vi "Initialize Channel Browser_Trigger.vi"(8 "error in (no error)":errorcluster, 9 "Trigger Parameters":T1, 10 ".NET Refnum in":refnum<k24>, 11 "Item Ref in":T2 format="%.0x") -> (0 "error out":errorcluster, 2 "Event":refnum<user-event>, 3 "Item Ref out":T2 format="%.0x")   [LabVIEW 2018, in "Instrument Addon System Explorer.lvlib"]
uses:
  Instrument Addon System Explorer.lvlib
  <vilib>/NI VeriStand/Custom Device Tools/Custom Device Utility Library/Custom Device Utility Library.lvlib
  <vilib>/NI VeriStand/Custom Device API/Custom Device API.lvlib
  NationalInstruments.VeriStand.SystemStorage
  NationalInstruments.VeriStand.SystemStorageUI
  <vilib>/NI VeriStand/UI Controls/Single Node Browser/NI_VS UI Single Node Browser.lvlib
  NationalInstruments.VeriStand
  Addon Shared/SubVIs/Constants.vi
  Addon Shared/Instrument Addon Shared.lvlib
  <vilib>/NI VeriStand/Custom Device API/Custom Device Item Ref.ctl
  <vilib>/NI VeriStand/UI Controls/Single Node Browser/Net Event.ctl
  <vilib>/NI VeriStand/UI Controls/Single Node Browser/Net Event Data.ctl
  Addon Shared/Types/Trigger Parameters.ctl
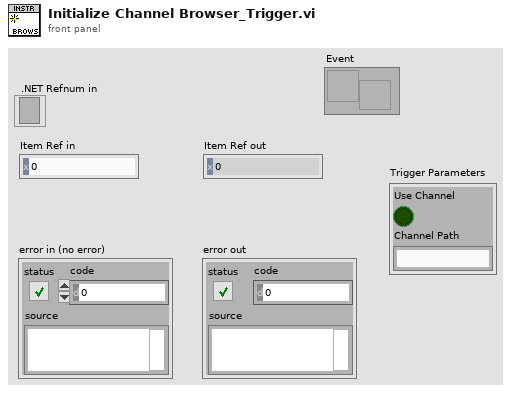
[diagram p1: front panel]
types:
  T1 = typedef "Instrument Addon Shared.lvlib/Trigger Parameters.ctl" = cluster{"Use Channel":bool, "Channel Path":string}
  T2 = typedef "Custom Device API.lvlib/Custom Device Item Ref.ctl" = u64
  T3 = typedef "Custom Device API.lvlib/Custom Device Pointer.ctl" = refnum<k24>
  T4 = typedef "NI_VS UI Single Node Browser.lvlib/Callback Type.ctl" = cluster{"Net Callbacks":refnum<k27>[], "Event":refnum<user-event>}
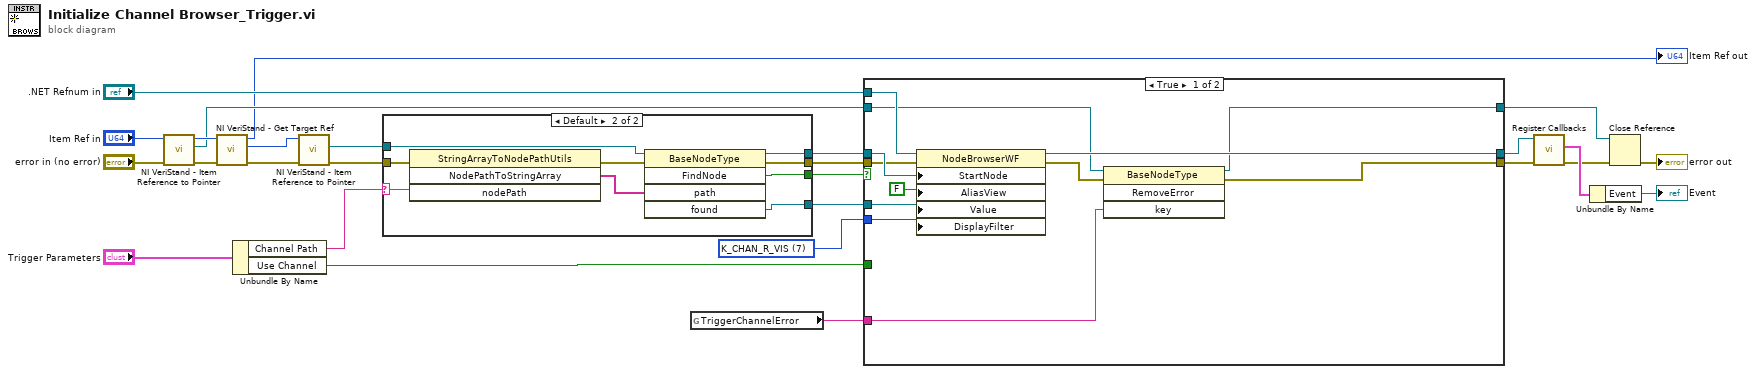
[diagram p0: block diagram]
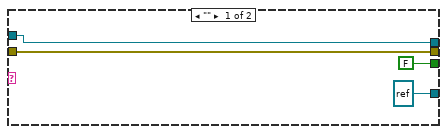
[diagram p2: hidden frame]
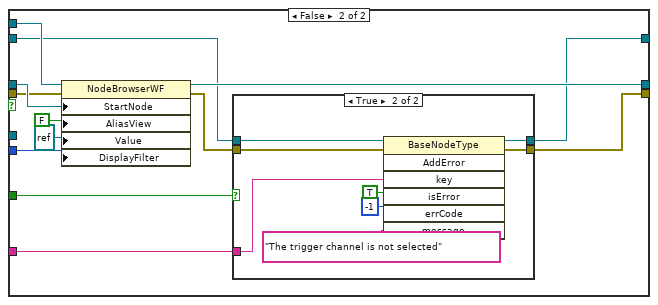
[diagram p3: hidden frame]
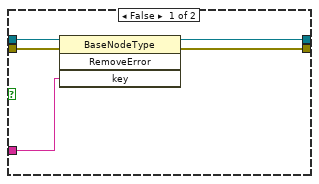
[diagram p4: hidden frame]
diagram:
  w26 = u8 7 items=["K_CHAN_R", "K_CHAN_W", "K_CHAN_RW", "K_CHAN_VOLT", "K_CHAN_FAULT", "K_ALL", "K_CUSTOM", "K_CHAN_R_VIS", "K_CHAN_W_VIS", "K_CHAN_RW_VIS", "K_CHAN_VOLT_VIS", "K_CHAN_FAULT_VIS"] ("DisplayFilter")
  n1 = call <vilib>:"NI VeriStand - Item Reference to Pointer.vi"("error in (no error)"="error in (no error)", "Item Ref in"="Item Ref in") -> ("error out"=w9:errorcluster, "Node Pointer"=w6:T3, "Item Ref out"=w7:T2)  [unwired: 6 in, 1 out]
  n2 = call <vilib>:"NI VeriStand - Get Target Ref.vi"("error in"=w9, "Item Ref in"=w7) -> ("error out"=w27:errorcluster, "Target Ref"=w20:T2, "Item Ref out"=→"Item Ref out":T2)  [unwired: 6 in, 1 out]
  n3 = Unbundle By Name("Trigger Parameters") -> ("Channel Path"=w12:string, "Use Channel"=w11:bool)
  n4 = call <vilib>:"NI VeriStand - Item Reference to Pointer.vi"("error in (no error)"=w27, "Item Ref in"=w20) -> ("error out"=w22:errorcluster, "Node Pointer"=w21:T3)  [unwired: 6 in, 2 out]
  n5 = case shown="Default" w12 {
    selector: w12 -> [_ w33]
    tunnel: [refnum<k24> refnum ("Value") w40] -> w25
    tunnel: [w30 w39] -> w24
    tunnel: [w31 w38] -> w23
    tunnel: w22 -> [w31 w36]
    tunnel: w21 -> [w30 w35]
    tunnel: [FALSE ("FindNode") w34] -> w19
    frame "" {
    }
    frame Default {
      n6 = invoke class="StringArrayToNodePathUtils" method="NodePathToStringArray"(error in=w36, "nodePath"=w33) -> (error out=w37:errorcluster, "NodePathToStringArray"=w32:string[])  [unwired: 2 in, 2 out]
      n7 = invoke class="BaseNodeType" method="FindNode"(reference=w35, error in=w37, "path"=w32) -> (reference out=w39:T3, error out=w38:errorcluster, "FindNode"=w34:bool, "found"=w40:refnum<k24>)  [unwired: 2 in, 1 out]
    }
  }
  n8 = global read "Constants.vi" "TriggerChannelError"() -> (w1:string)
  n9 = case shown="True" w19 {
    tunnel: w26 -> [w48 w60]
    tunnel: ".NET Refnum in" -> [w52 w65]
    tunnel: [w44 w57] -> w16
    tunnel: w24 -> [w51 w64]
    tunnel: w23 -> [w50 w63]
    tunnel: w25 -> [w49 _]
    tunnel: [w46 w62] -> w15
    tunnel: w11 -> [_ w56]
    tunnel: w6 -> [w43 w55]
    tunnel: [w42 w54] -> w4
    tunnel: w1 -> [w41 w53]
    frame True {
      n10 = property class="NodeBrowserWF"(reference=w52, error in=w50, "StartNode"=w51, "AliasView"=FALSE, "Value"=w49, "DisplayFilter"=w48) -> (reference out=w46:refnum<k24>, error out=w45:errorcluster)
      n11 = invoke class="BaseNodeType" method="RemoveError"(reference=w43, error in=w45, "key"=w41) -> (reference out=w42:T3, error out=w44:errorcluster)  [unwired: 1 in, 2 out]
    }
    frame False {
      n12 = property class="NodeBrowserWF"(reference=w65, error in=w63, "StartNode"=w64, "AliasView"=FALSE, "Value"=refnum<k24> refnum, "DisplayFilter"=w60) -> (reference out=w62:refnum<k24>, error out=w58:errorcluster)
      n13 = case shown="True" w56 {
        tunnel: w58 -> [w70 w74]
        tunnel: [w69 w78] -> w57
        tunnel: w55 -> [w68 w75]
        tunnel: [w67 w72] -> w54
        tunnel: w53 -> [w66 w71]
        frame False {
          n14 = invoke class="BaseNodeType" method="RemoveError"(reference=w68, error in=w70, "key"=w66) -> (reference out=w67:T3, error out=w69:errorcluster)  [unwired: 1 in, 2 out]
        }
        frame True {
          n15 = invoke class="BaseNodeType" method="AddError"(reference=w75, error in=w74, "key"=w71, "isError"=TRUE, "errCode"=-1, "message"="The trigger channel is not selected") -> (reference out=w72:T3, error out=w78:errorcluster)  [unwired: 1 in, 5 out]
        }
      }
    }
  }
  n16 = call <vilib>:"Register Callbacks.vi"("error in (no error)"=w16, "Single Node Browser"=w15) -> ("error out"=w3:errorcluster, "Callbacks"=w18:T4)  [unwired: 7 in, 1 out]
  n17 = Unbundle By Name(w18) -> ("Event"=→"Event":refnum<user-event>)
  n18 = Close Reference(reference=w4, error in (no error)=w3) -> (error out=→"error out":errorcluster)
